vi "RP hoekcorrelatie-analyse.vi"() -> ()   [LabVIEW 2013]
uses:
  Instance           8 17Saved   practicum .vi
  Instance          13 17Saved   practicum .vi
  Instance          11 17Saved   practicum .vi
  Instance          10 17Saved   practicum .vi
  Instance          12 17Saved   practicum .vi
  Instance           5 17Saved   practicum .vi
  Instance           3 17Saved   practicum .vi
  Instance           9 17Saved   practicum .vi
  Instance           7 17Saved   practicum .vi
  Instance           2 17Saved   practicum .vi
  Instance           1 17Saved   practicum .vi
  Instance           6 17Saved   practicum .vi
  Instance           4 17Saved   practicum .vi
  <vilib>/Utility/file.llb/Read From Spreadsheet File (DBL).vi
panel:
  in  "sigma (mrad) 2":dbl
  out "Sum of squared residuals":dbl
  out "output cluster 2":cluster{ext[], ext[]}
  out "XY Graph 5":cluster{ext[], ext[]}[](graph)
  out "2d - Acar 4":bool
  out "2d - Acar 3":bool
  out "Numeric":dbl
  out "2d - Acar 2":bool
  in  "1d - Acar":bool caption="2d - Acar or DB"
  out "?":dbl format="%#_3g"
  in  "22Na source radius (mm)":dbl=0.1 min=1e-05 max=3.0
  in  "measurement file\n\n         ??. txt":bool
  out "Fermi energy (eV)":dbl format="%#_3g"
  out "Numeric 5":dbl format="%#_3g"
  out "Numeric 4":dbl format="%#_3g"
  out "Numeric 3":dbl format="%#_3g"
  out "Numeric 2":dbl format="%#_3g"
  in  "background \n coincidence counts":dbl min=0.0 max=100.0
  in  "alignment correction":dbl min=-10.0 max=10.0 step=0.0001
  out "XY Graph 4":cluster{ext[], ext[]}[](graph)
  in  "stop 4":bool
  in  "collimator afstand\n       (mm)":dbl=500.0 min=100.0 max=1000.0
  in  "spleetbreedte\n      (mm)":dbl=1.0 min=0.1 max=5.0
  out "ZICHT  functie":cluster{"Y":dbl[], "Y":dbl[]}[](graph)
  out "?":dbl format="%#_3g"
  in  "fraction core\nannihilations":dbl=0.2 min=0.0 max=1.0 step=1e-05
  in  "core width\n   (mrad)":dbl=5.0
  out "core electrons":cluster{"Y":dbl[], "Y":dbl[]}[](graph)
  in  "stop 2":bool
  in  "Fermi angle\n   (mrad)":dbl=7.0
  out "free gas model":cluster{"Y":dbl[], "Y":dbl[]}[](graph)
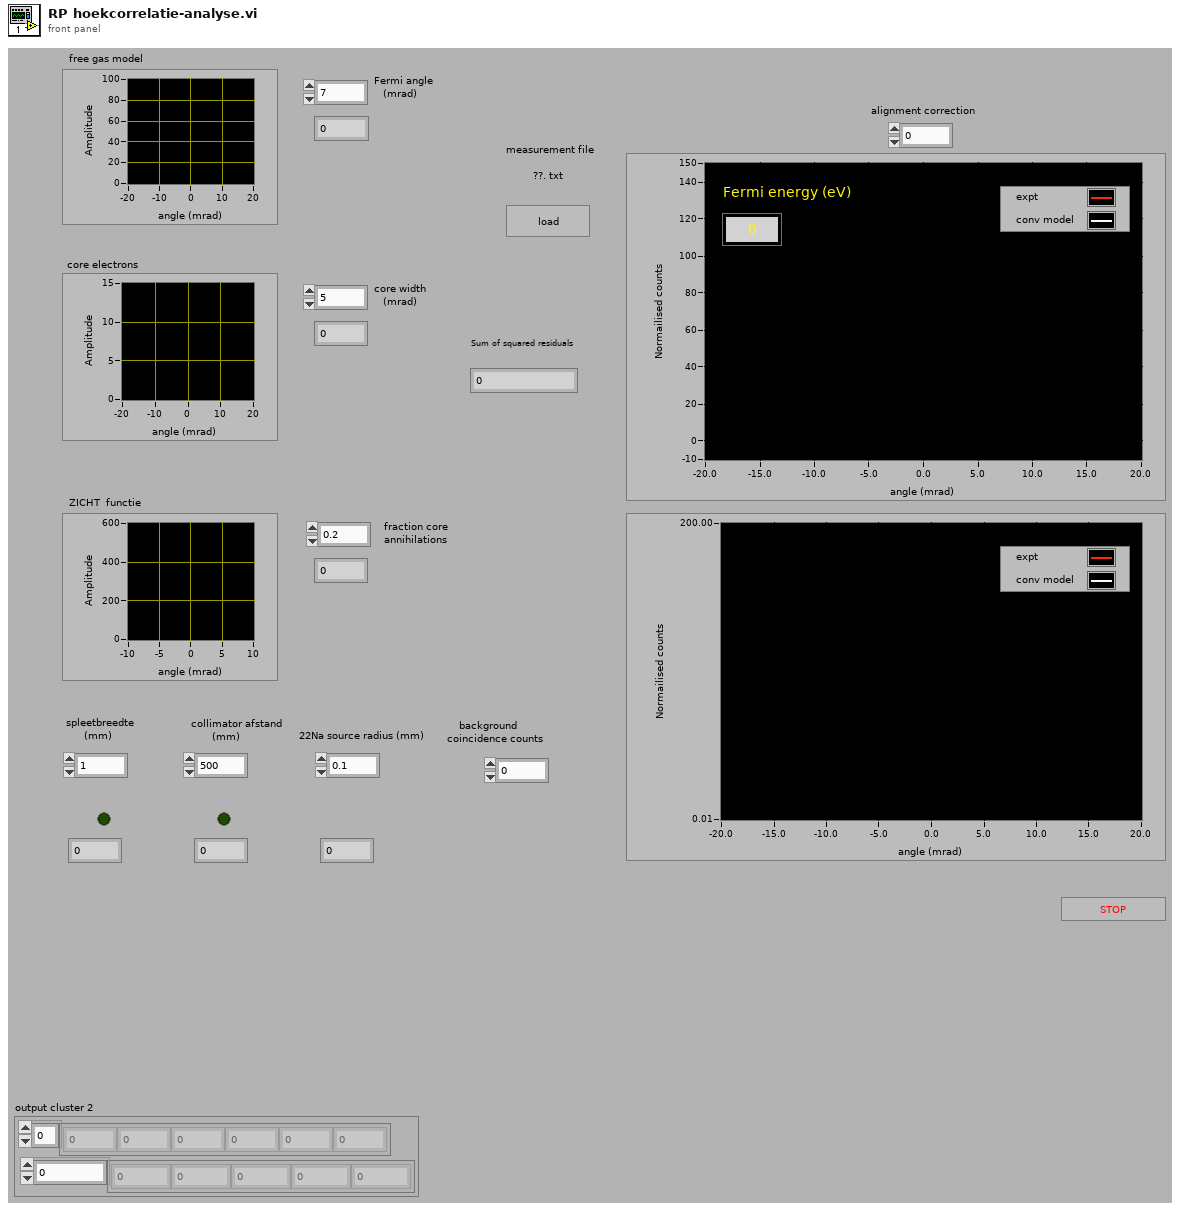
[diagram p1: front panel]
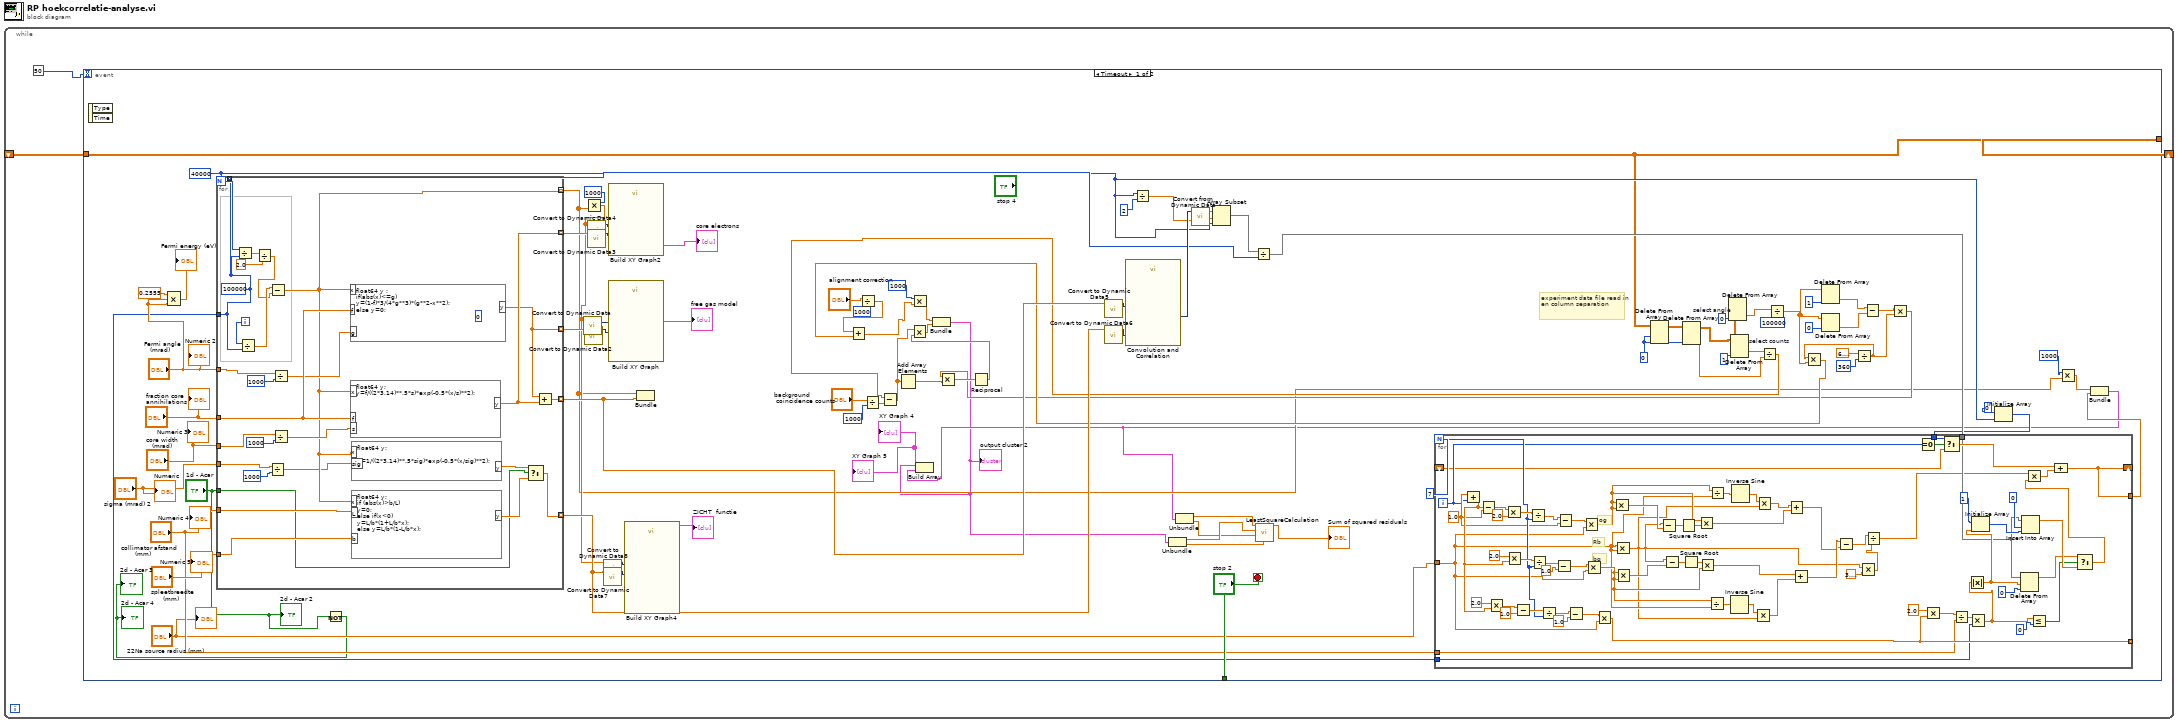
[diagram p0: block diagram]
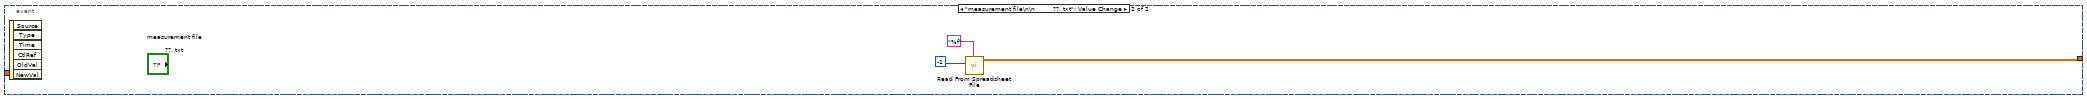
[diagram p2: hidden frame]
diagram:
  n1 = while {
    shift-right: [w2] -> _
    shift-left: _ -> [w1]
    stop <- w4 stop-if-true
    n2 = event shown="[0] Timeout" {
      selector: _ -> [_ _]
      dyn-events: _ -> [_ _]
      timeout: 50 -> [_ _]
      tunnel: ["stop 2" _] -> w4
      tunnel: [w16 w191] -> w2
      tunnel: w1 -> [w16 _]
      event Timeout {
        w49 = 0
        w32 = 40000
        # "experiment data file read in\nen column separation"
        n3 = event-data() -> ()  [unwired: 1 in, 2 out]
        n4 = Compound Arithmetic op=MULTIPLY(0.2555, "Fermi angle\n   (mrad)", "Fermi angle\n   (mrad)") -> (→"Fermi energy (eV)":dbl)
        n5 = for {
          N: w32 -> [w184]
          tunnel: [w166] -> w17 mode=indexing
          tunnel: [w173] -> w90 mode=indexing
          tunnel: "Fermi angle\n   (mrad)" -> [w183]
          tunnel: [w177] -> w87 mode=indexing
          tunnel: "core width\n   (mrad)" -> [w181]
          tunnel: "fraction core\nannihilations" -> [w175]
          tunnel: [w179] -> w55 mode=indexing
          tunnel: "spleetbreedte\n      (mm)" -> [w171]
          tunnel: "collimator afstand\n       (mm)" -> [w172]
          tunnel: [w178] -> w58 mode=indexing
          tunnel: [w170] -> w56 mode=indexing
          tunnel: [w178] -> w34
          tunnel: "1d - Acar" -> [w167]
          tunnel: "sigma (mrad) 2" -> [w164]
          i -> [w188]
          (unwired) 0
          w178 = 100000
          # "gauss"
          # "parabool"
          # "tentfunctie"
          n6 = Divide(x=w184, y=w178) -> (x/y=w187:dbl)
          n7 = Divide(x=w188, y=w178) -> (x/y=w189:dbl)
          n8 = Divide(x=w187, y=2.0) -> (x/y=w185:dbl)
          n9 = Divide(x=w164, y=1000) -> (x/y=w163:dbl)
          n10 = Subtract(x=w189, y=w185) -> (x-y=w166:dbl)
          n11 = Divide(x=w183, y=1000) -> (x/y=w174:dbl)
          n12 = Divide(x=w181, y=1000) -> (x/y=w176:dbl)
          n13 = formula code="float64 y ;\nif(abs(x)<=g)\ny=(1-f)*3/(4*g**3)*(g**2-x**2);\nelse y=0;"("x"=w166, "g"=w174, "f"=w175) -> ("y"=w173:dbl)
          n14 = formula code="float64 y;\ny=f/((2*3.14)**.5*s)*exp(-0.5*(x/s)**2);"("x"=w166, "s"=w176, "f"=w175) -> ("y"=w177:dbl)
          n15 = formula code="float64 y;\n\ny=1/((2*3.14)**.5*sig)*exp(-0.5*(x/sig)**2);"("x"=w166, "sig"=w163) -> ("y"=w169:dbl)
          n16 = formula code="float64 y;\nif (abs(x)>b/L)\ny=0;\nelse if(x<0)\ny=L/b*(1+L/b*x);\nelse y=L/b*(1-L/b*x);"("x"=w166, "b"=w171, "L"=w172) -> ("y"=w168:dbl)
          n17 = Select(t=w169, s=w167, f=w168) -> (s? t:f=w170:dbl)
          n18 = Add(x=w173, y=w177) -> (x+y=w179:dbl)
        }
        n19 = Not(x="1d - Acar") -> (.not. x?=→"2d - Acar 3" →"2d - Acar 4":bool)
        n20 = call "Convert to Dynamic Data2"("Array"=w90) -> ("Dynamic Data Type"=w92:dynamicdata)  [unwired: 3 in]
        n21 = Multiply(x=1000, y=w17) -> (x*y=w26:dbl[])
        n22 = call "Convert to Dynamic Data"("Array"=w26) -> ("Dynamic Data Type"=w91:dynamicdata)  [unwired: 3 in]
        n23 = call "Convert to Dynamic Data4"("Array"=w26) -> ("Dynamic Data Type"=w85:dynamicdata)  [unwired: 3 in]
        n24 = call "Convert to Dynamic Data3"("Array"=w87) -> ("Dynamic Data Type"=w86:dynamicdata)  [unwired: 3 in]
        n25 = call "Convert to Dynamic Data8"("Array"=w26) -> ("Dynamic Data Type"=w81:dynamicdata)  [unwired: 3 in]
        n26 = call "Convert to Dynamic Data7"("Array"=w56) -> ("Dynamic Data Type"=w82:dynamicdata)  [unwired: 3 in]
        n27 = call "Build XY Graph2"("Y Input"=w86, "X Input"=w85) -> ("XY Graph"=→"core electrons":cluster{"Y":dbl[], "Y":dbl[]}[])  [unwired: 8 in, 1 out]
        n28 = call "Build XY Graph"("Y Input"=w92, "X Input"=w91) -> ("XY Graph"=→"free gas model":cluster{"Y":dbl[], "Y":dbl[]}[])  [unwired: 8 in, 1 out]
        n29 = call "Build XY Graph4"("Y Input"=w82, "X Input"=w81) -> ("XY Graph"=→"ZICHT  functie":cluster{"Y":dbl[], "Y":dbl[]}[])  [unwired: 8 in, 1 out]
        n30 = Bundle(w17, w55) -> ()  [unwired: 1 in, 1 out]
        n31 = Divide(x="alignment correction", y=1000) -> (x/y=w79:dbl)
        n32 = Divide(x="background \n coincidence counts", y=1000) -> (x/y=w77:dbl)
        n33 = call "Convert to Dynamic Data5"("Array"=w55) -> ("Dynamic Data Type"=w64:dynamicdata)  [unwired: 3 in]
        n34 = call "Convert to Dynamic Data6"("Array"=w56) -> ("Dynamic Data Type"=w57:dynamicdata)  [unwired: 3 in]
        n35 = call "Convolution and Correlation"("Y"=w57, "X"=w64) -> ("X*Y"=w63:dynamicdata)  [unwired: 8 in, 1 out]
        n36 = Divide(x=w32, y=2) -> (x/y=w59:dbl)
        n37 = call "Convert from Dynamic Data"("Dynamic Data Type"=w63) -> ("Array"=w62:dbl[])  [unwired: 3 in]
        n38 = Array Subset(array=w62, index=w59, length=w32) -> (w61:dbl[])
        n39 = Divide(x=w61, y=w58) -> (x/y=w31:dbl[])
        n40 = Delete From Array(array=w16, index (row)=w49) -> (array with subset deleted=w52:ext[][])  [unwired: 2 in, 1 out]
        n41 = Delete From Array(array=w52, index (col)=w49) -> (deleted portion=w48:ext[], array with subset deleted=w51:ext[][])  [unwired: 2 in]
        n42 = Delete From Array "select angle"(array=w51, index (col)=0) -> (deleted portion=w14:ext[])  [unwired: 2 in, 1 out]
        n43 = Delete From Array "select counts"(array=w51, index (col)=1) -> (deleted portion=w50:ext[])  [unwired: 2 in, 1 out]
        n44 = Divide(x=w50, y=w48) -> (x/y=w38:ext[])
        n45 = Subtract(x=w38, y=w77) -> (x-y=w73:ext[])
        n46 = Add Array Elements(numeric array=w73) -> (sum=w72:ext)
        n47 = Divide(x=w14, y=100000) -> (x/y=w13:ext[])
        n48 = Delete From Array(array=w13, index=1) -> (deleted portion=w45:ext)  [unwired: 1 in, 1 out]
        n49 = Delete From Array(array=w13, index=0) -> (deleted portion=w44:ext)  [unwired: 1 in, 1 out]
        n50 = Divide(x=6.283185307179586, y=360) -> (x/y=w40:dbl)
        n51 = Multiply(x=w40, y=w13) -> (x*y=w39:ext[])
        n52 = Add(x=w79, y=w39) -> (x+y=w24:ext[])
        n53 = Multiply(x=1000, y=w24) -> (x*y=w25:ext[])
        n54 = Subtract(x=w45, y=w44) -> (x-y=w41:ext)
        n55 = Multiply(x=w41, y=w40) -> (x*y=w37:ext)
        n56 = Multiply(x=w37, y=w72) -> (x*y=w71:ext)
        n57 = Reciprocal(x=w71) -> (1/x=w70:ext)
        n58 = Multiply(x=w73, y=w70) -> (x*y=w74:ext[])
        n59 = Bundle(w25, w74) -> (w11:cluster{ext[], ext[]})  [unwired: 1 in]
        "output cluster 2" <- w11
        n60 = Unbundle(w11) -> (w8:ext[], w6:ext[])
        n61 = Initialize Array(0, w32) -> (w30:i32[])
        n62 = for {
          N: 7 -> [w148]
          tunnel: "22Na source radius (mm)" -> [w132]
          tunnel: [w118] -> _ mode=indexing
          tunnel: "collimator afstand\n       (mm)" -> [w116]
          tunnel: w34 -> [w115]
          tunnel: w31 -> [w101]
          tunnel: w30 -> [w99]
          shift-right: [w97] -> _
          shift-left: _ -> [w98]
          tunnel: [w97] -> w28
          i -> [w100]
          w143 = 1.0 ("x")
          # "Rb"
          # "bg"
          # "og"
          n63 = Add(x=w143, y=w100) -> (x+y=w144:dbl)
          n64 = Subtract(x=w144, y=w143) -> (x-y=w161:dbl)
          n65 = Multiply(x=2.0, y=w144) -> (x*y=w151:dbl)
          n66 = Multiply(x=w161, y=2.0) -> (x*y=w160:dbl)
          n67 = Multiply(x=2.0, y=w144) -> (x*y=w156:dbl)
          n68 = Subtract(x=w151, y=1.0) -> (x-y=w149:dbl)
          n69 = Divide(x=w160, y=w148) -> (x/y=w159:dbl)
          n70 = Divide(x=w156, y=w148) -> (x/y=w155:dbl)
          n71 = Divide(x=w149, y=w148) -> (x/y=w147:dbl)
          n72 = Subtract(x=w155, y=1.0) -> (x-y=w153:dbl)
          n73 = Subtract(x=w159, y=w143) -> (x-y=w158:dbl)
          n74 = Subtract(x=w147, y=1.0) -> (x-y=w145:dbl)
          n75 = Multiply(x=w158, y=w132) -> (x*y=w133:dbl)
          n76 = Multiply(x=w153, y=w132) -> (x*y=w136:dbl)
          n77 = Multiply(x=w145, y=w132) -> (x*y=w118:dbl)
          n78 = Multiply(x=w133, y=w133) -> (x*y=w139:dbl)
          n79 = Multiply(x=w132, y=w132) -> (x*y=w122:dbl)
          n80 = Multiply(x=w136, y=w136) -> (x*y=w142:dbl)
          n81 = Subtract(x=w122, y=w139) -> (x-y=w138:dbl)
          n82 = Subtract(x=w122, y=w142) -> (x-y=w141:dbl)
          n83 = Square Root(x=w138) -> (sqrt(x)=w137:dbl)
          n84 = Square Root(x=w141) -> (sqrt(x)=w140:dbl)
          n85 = Multiply(x=w133, y=w137) -> (x*y=w126:dbl)
          n86 = Multiply(x=w140, y=w136) -> (x*y=w129:dbl)
          n87 = Divide(x=w136, y=w132) -> (x/y=w135:dbl)
          n88 = Divide(x=w133, y=w132) -> (x/y=w131:dbl)
          n89 = Inverse Sine(1:w135) -> (0:w134:dbl)
          n90 = Inverse Sine(1:w131) -> (0:w130:dbl)
          n91 = Multiply(x=w134, y=w122) -> (x*y=w128:dbl)
          n92 = Multiply(x=w130, y=w122) -> (x*y=w127:dbl)
          n93 = Add(x=w127, y=w126) -> (x+y=w124:dbl)
          n94 = Add(x=w129, y=w128) -> (x+y=w125:dbl)
          n95 = Subtract(x=w125, y=w124) -> (x-y=w121:dbl)
          n96 = Multiply(x=w122, y=3.141592653589793) -> (x*y=w120:dbl)
          n97 = Divide(x=w121, y=w120) -> (x/y=w94:dbl)
          n98 = Equal To 0?(x=w100) -> (x = 0?=w109:bool)
          n99 = Multiply(x=2.0, y=w118) -> (x*y=w117:dbl)
          n100 = Select(t=w99, s=w109, f=w98) -> (s? t:f=w108:dbl[])
          n101 = Divide(x=w117, y=w116) -> (x/y=w114:dbl)
          n102 = Multiply(x=w114, y=w115) -> (x*y=w104:dbl)
          n103 = Absolute Value(x=w104) -> (abs(x)=w103:dbl)
          n104 = Initialize Array(1, w103) -> (w111:i32[])
          n105 = Delete From Array(array=w101, length=w103, index=0) -> (array with subset deleted=w106:dbl[])  [unwired: 1 out]
          n106 = Insert Into Array(array=w101, index=0, new element=w111) -> (w107:dbl[])
          n107 = Less Or Equal?(x=w104, y=0) -> (x <= y?=w102:bool)
          n108 = Select(t=w106, s=w102, f=w107) -> (s? t:f=w95:dbl[])
          n109 = Multiply(x=w94, y=w95) -> (x*y=w96:dbl[])
          n110 = Compound Arithmetic op=ADD(w108, w96) -> (w97:dbl[])
        }
        n111 = Multiply(x=1000, y=w17) -> (x*y=w21:dbl[])
        n112 = Bundle(w21, w28) -> (w12:cluster{dbl[], dbl[]})  [unwired: 1 in]
        n113 = Build Array(w11, w12) -> (→"XY Graph 4" →"XY Graph 5":cluster{ext[], ext[]}[])
        n114 = Unbundle(w12) -> (w9:dbl[], w7:dbl[])
        n115 = call "LeastSquareCalculation.vi"("array 4"=w6, "array 3"=w7, "array 2"=w8, "array"=w9) -> ("Numeric"=→"Sum of squared residuals":dbl)  [unwired: 7 in]
        "?" <- "fraction core\nannihilations"
        "Numeric 2" <- "Fermi angle\n   (mrad)"
        "Numeric 3" <- "core width\n   (mrad)"
        "Numeric 4" <- "collimator afstand\n       (mm)"
        "Numeric 5" <- "spleetbreedte\n      (mm)"
        "?" <- "22Na source radius (mm)"
        "2d - Acar 2" <- "1d - Acar"
        "Numeric" <- "sigma (mrad) 2"
      }
      event "measurement file\n\n         ??. txt": Value Change {
        n116 = event-data() -> ()  [unwired: 1 in, 6 out]
        n117 = call-poly <vilib>:"Read From Spreadsheet File.vi"("format (%.3f)"="%f", "number of rows (all:-1)"=-1) -> ("all rows"=w191:ext[][])  [unwired: 5 in, 4 out]
      }
    }
  }
